vi "Close VI Reference.vi"(8 "error in (no error)":errorcluster, 10 "VI Refnum":refnum<vi>, 11 "Plugin Server in":refnum<class "Generic Plugin.lvclass">) -> (0 "error out":errorcluster, 2 "Reference was already closed":bool, 3 "Plugin Server out":refnum<class "Generic Plugin.lvclass">)   [LabVIEW 2020, in "RxnRover.lvlib" / "Generic Plugin.lvclass"]
doc: "Closes a VI reference. This VI is intented to work both in the development environment and in stand-alone programs."
uses:
  Generic Plugin.lvclass
  Generic Plugin.lvclass/Generic Plugin.ctl
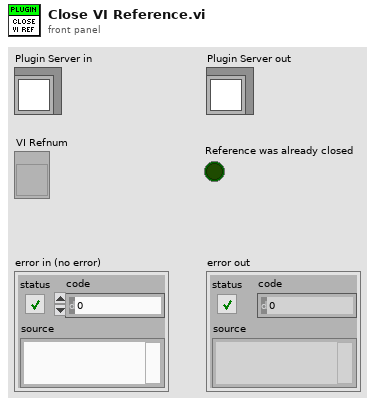
[diagram p1: front panel]
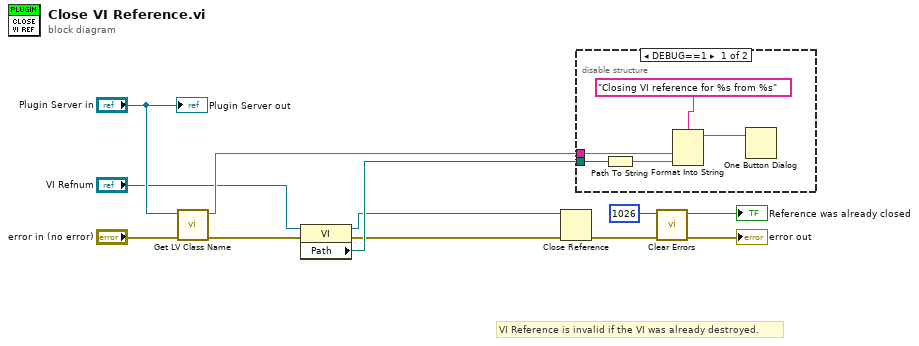
[diagram p0: block diagram]
diagram:
  # "VI Reference is invalid if the VI was already destroyed."
  n1 = call <vilib>:"Get LV Class Name.vi"("error in (no error)"="error in (no error)", "object"="Plugin Server in") -> ("error out"=w7:errorcluster, "class name"=w12:string)  [unwired: 8 in]
  n2 = property class="VI"(reference="VI Refnum", error in=w7) -> (reference out=w5:refnum<vi>, error out=w6:errorcluster, "Path"=w8:path)
  n3 = Close Reference(reference=w5, error in (no error)=w6) -> (error out=w3:errorcluster)
  n4 = disable-structure shown="DEBUG==1" {
    disable-tunnel: w8 -> [w17 _]
    disable-tunnel: w12 -> [w13 _]
    frame condition #0 (active) {
      n5 = Path To String(path=w17) -> (string=w14:string)
      n6 = Format Into String(format string="Closing VI reference for %s from %s", w13, w14) -> (resulting string=w15:string)  [unwired: 2 in, 1 out]
      n7 = One Button Dialog(message=w15) -> ()  [unwired: 1 in, 1 out]
    }
    frame condition #1 {
      # "Do nothing"
    }
  }
  n8 = call <vilib>:"Clear Errors.vi"("error in (no error)"=w3, "specific error code to clear (0: all)"=1026) -> ("error out"=→"error out":errorcluster, "specific error cleared?"=→"Reference was already closed":bool)  [unwired: 4 in]
  "Plugin Server out" <- "Plugin Server in"
